vi "FunctDataMgr.Reference Qs.vi"(8 "error in (no error)":errorcluster, 9 "Q Local":refnum<queue>, 10 "Q Parent":refnum<queue>, 11 "FunctDataMgr in":refnum<class "FunctDataMgr.lvclass">) -> (0 "error out":errorcluster, 3 "FunctDataMgr":refnum<class "FunctDataMgr.lvclass">)   [LabVIEW 2018, in "FunctDataMgr.lvclass"]
uses:
  FunctDataMgr.lvclass
  <vilib>/KATE/Queues/Q.Element.ctl
  FunctDataMgr.lvclass/FunctDataMgr.ctl
  <vilib>/KATE/Queues/Queue Utils.lvlib
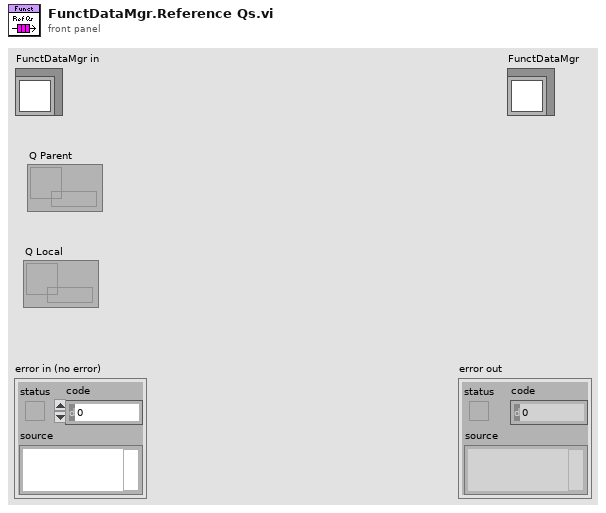
[diagram p1: front panel]
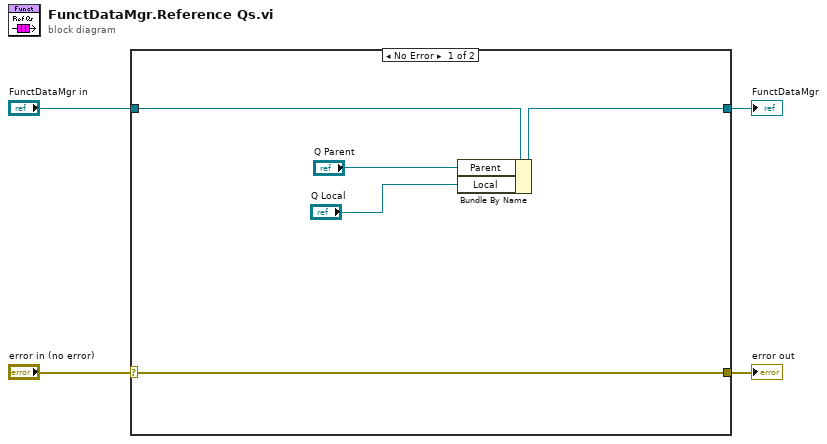
[diagram p0: block diagram]
diagram:
  n1 = case shown="No Error" "error in (no error)" {
    selector: "error in (no error)" -> [w9 w11]
    tunnel: [w9 w11] -> w3
    tunnel: [w7 w10] -> w1
    tunnel: "FunctDataMgr in" -> [w8 w10]
    frame No Error {
      n2 = Bundle By Name(cluster=w8, "Parent"="Q Parent", "Local"="Q Local") -> (w7:refnum<class "FunctDataMgr.lvclass">)
    }
    frame Error {
    }
  }
  "error out" <- w3
  "FunctDataMgr" <- w1
